vi "get vi name.vi"(8 "error in (no error)":errorcluster, 11 "vi ref":refnum<vi>) -> (0 "error out":errorcluster, 3 "vi name":string)   [LabVIEW 2024, in "status manager.lvlib"]
uses:
  status manager.lvlib
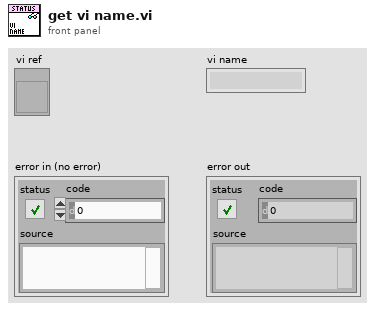
[diagram p1: front panel]
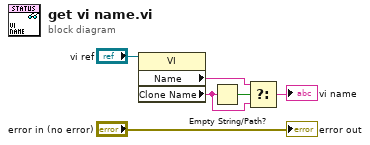
[diagram p0: block diagram]
diagram:
  n1 = property class="VI"(reference="vi ref") -> ("Name"=w2:string, "Clone Name"=w1:string)  [unwired: 1 in, 2 out]
  n2 = Empty String/Path?(string/path=w1) -> (empty?=w3:bool)
  n3 = Select(t=w2, s=w3, f=w1) -> (s? t:f=→"vi name":string)
  "error out" <- "error in (no error)"
